vi "HO6_Generator4.vi"() -> ()   [LabVIEW 2020]
panel:
  out "XY Graph":cluster{dbl[], dbl[]}(graph)
  out "Waveform Graph":waveform(dbl)[](graph)
  out "Exceed Low Threshold":bool
  out "Exceed High Threshold":bool
  out "High Threshold":dbl
  out "Low Threshold":dbl
  in  "stop":bool
  out "Strip Chart":T1(graph)
  in  "Max":dbl=500.0
  in  "Min":dbl=100.0
  out "When slope is >0, than it's green.":bool
  out "Current Overall average":dbl
  out "Biggest/Smallest value":T2 {"Big time" format="%<%.3X>T"}
  in  "Averaged Points":i16=5 min=1 max=1024 step=1
  in  "?":bool
  in  "Mode":bool
  out "?":enum32{"Iterations", "Timed"}(tab)
  out "Iterations Remaining":i32=15
  in  "Iterations to run":i32=10 min=1 step=1
  in  "Time to run (s)":dbl=15.0
  in  "Delay (ms)":i16=500
  out "Countdown (s)":dbl caption="Elapsed Time (s)"
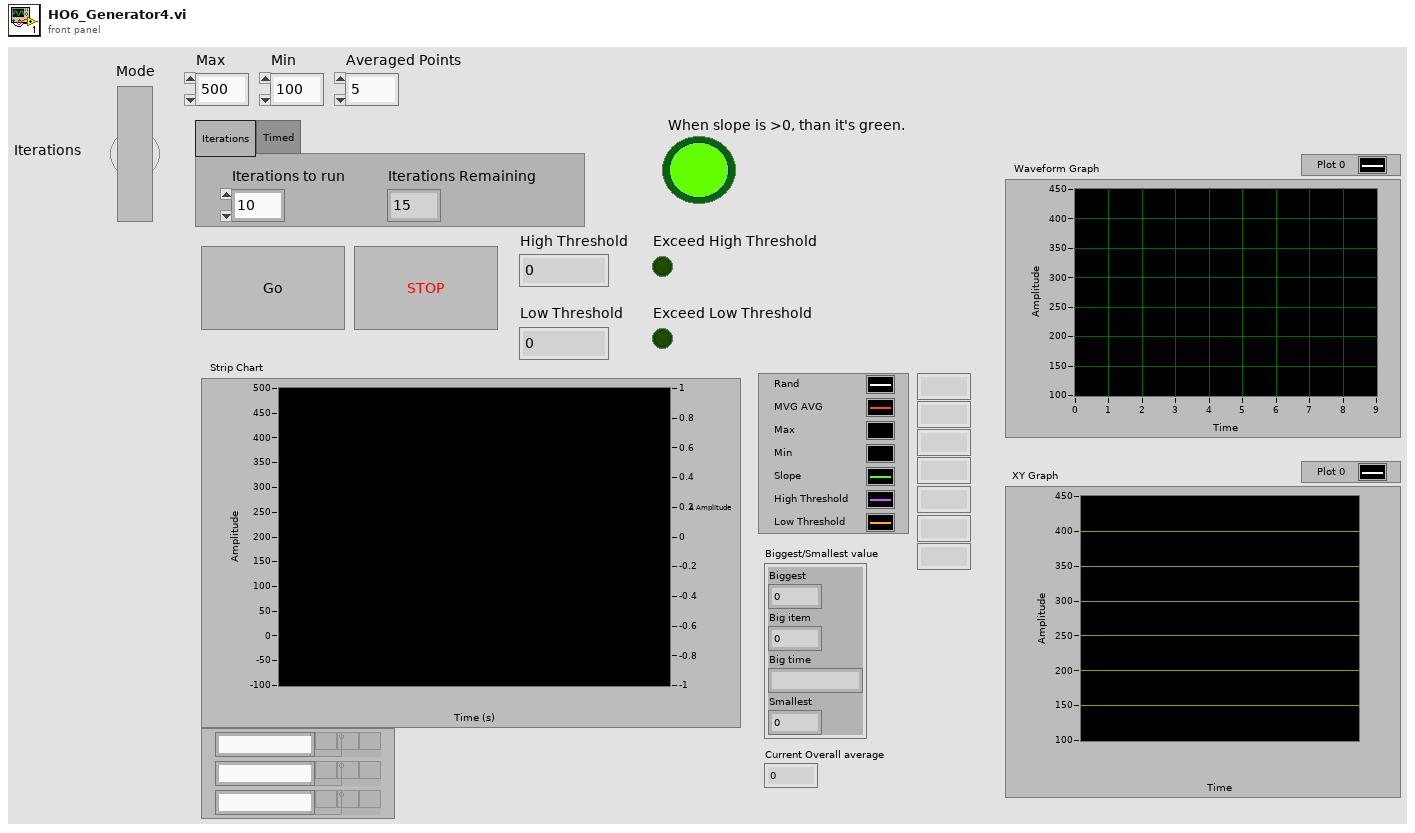
[diagram p1: front panel]
types:
  T1 = cluster{"Double":dbl, dbl, "Max":dbl, "Min":dbl, "Theta (degree)":dbl, dbl, dbl}
  T2 = cluster{"Biggest":dbl, "Big item":i32, "Big time":timestamp, "Smallest":dbl}
  T3 = cluster{"Double":dbl, dbl, "Max":dbl, "Min":dbl, "Theta (degree)":dbl, dbl, dbl}[]
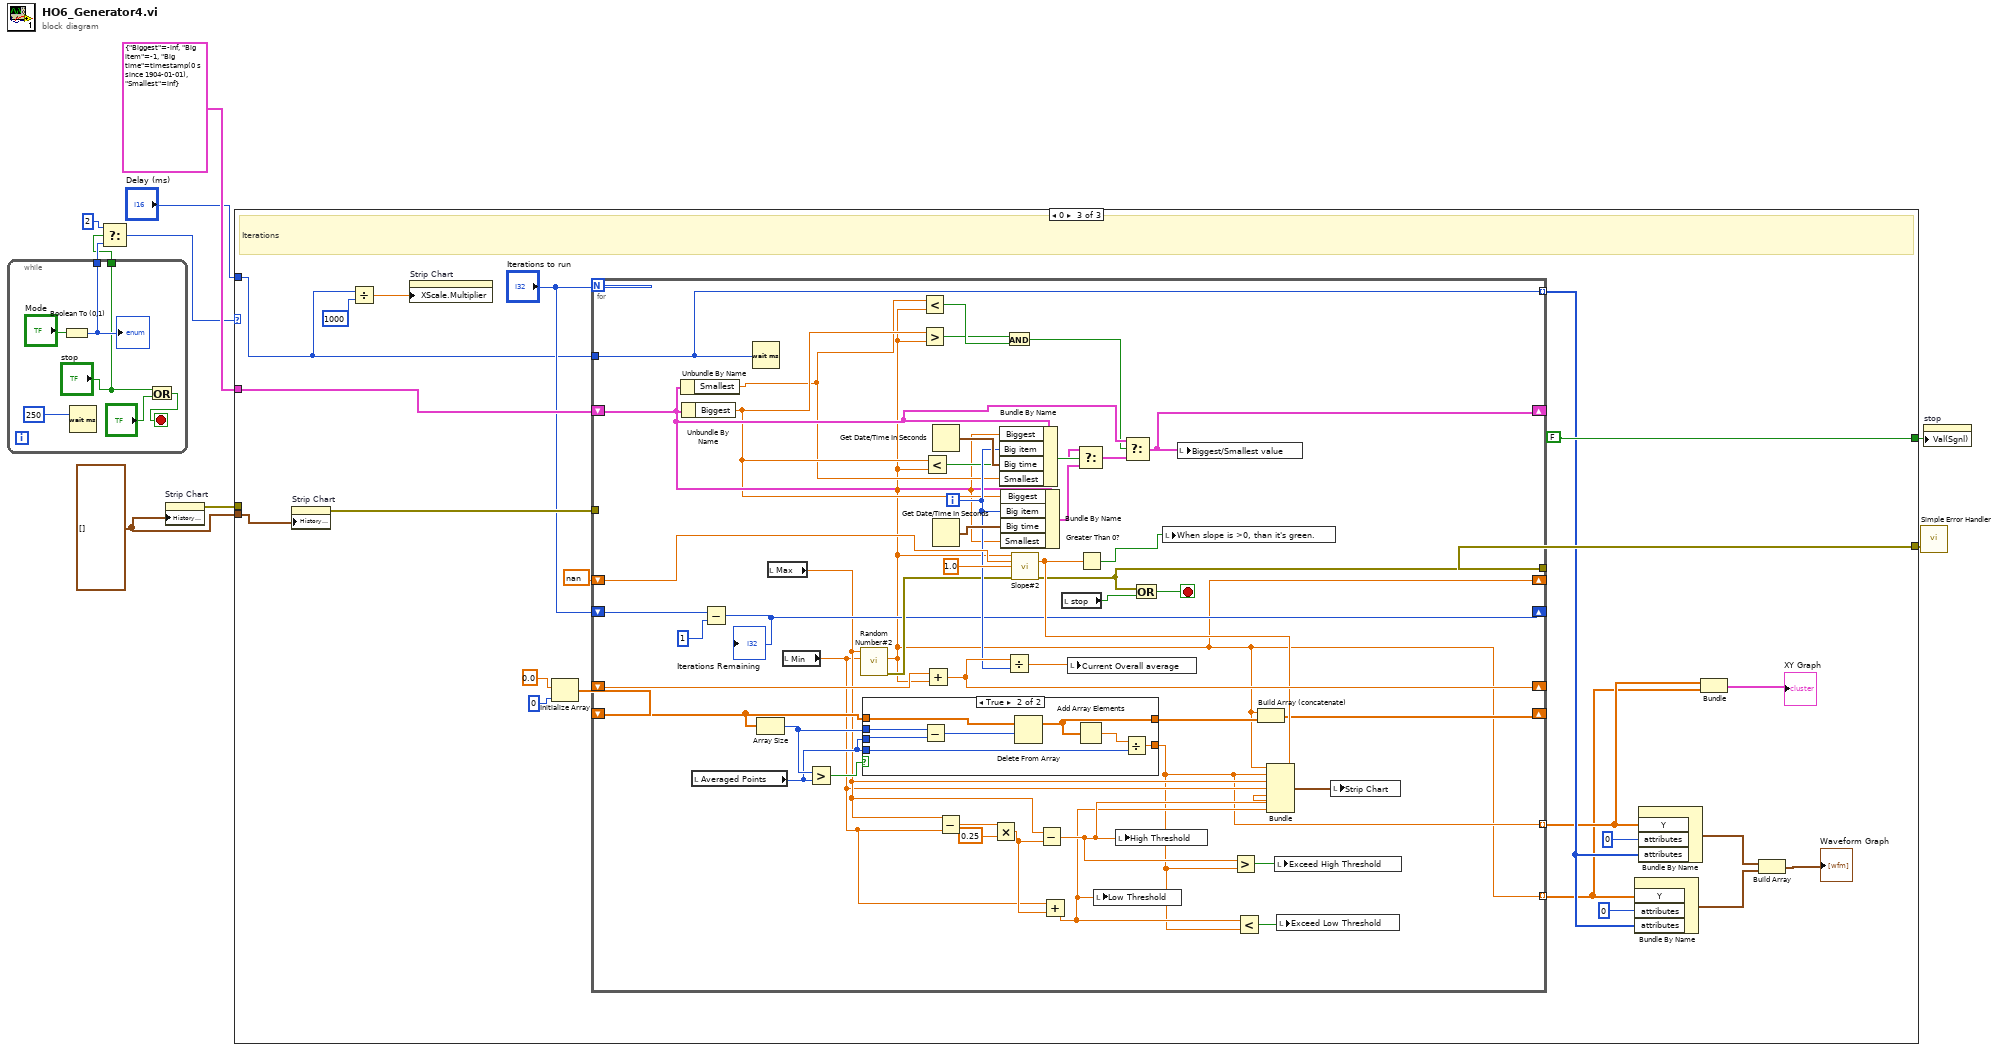
[diagram p0: block diagram]
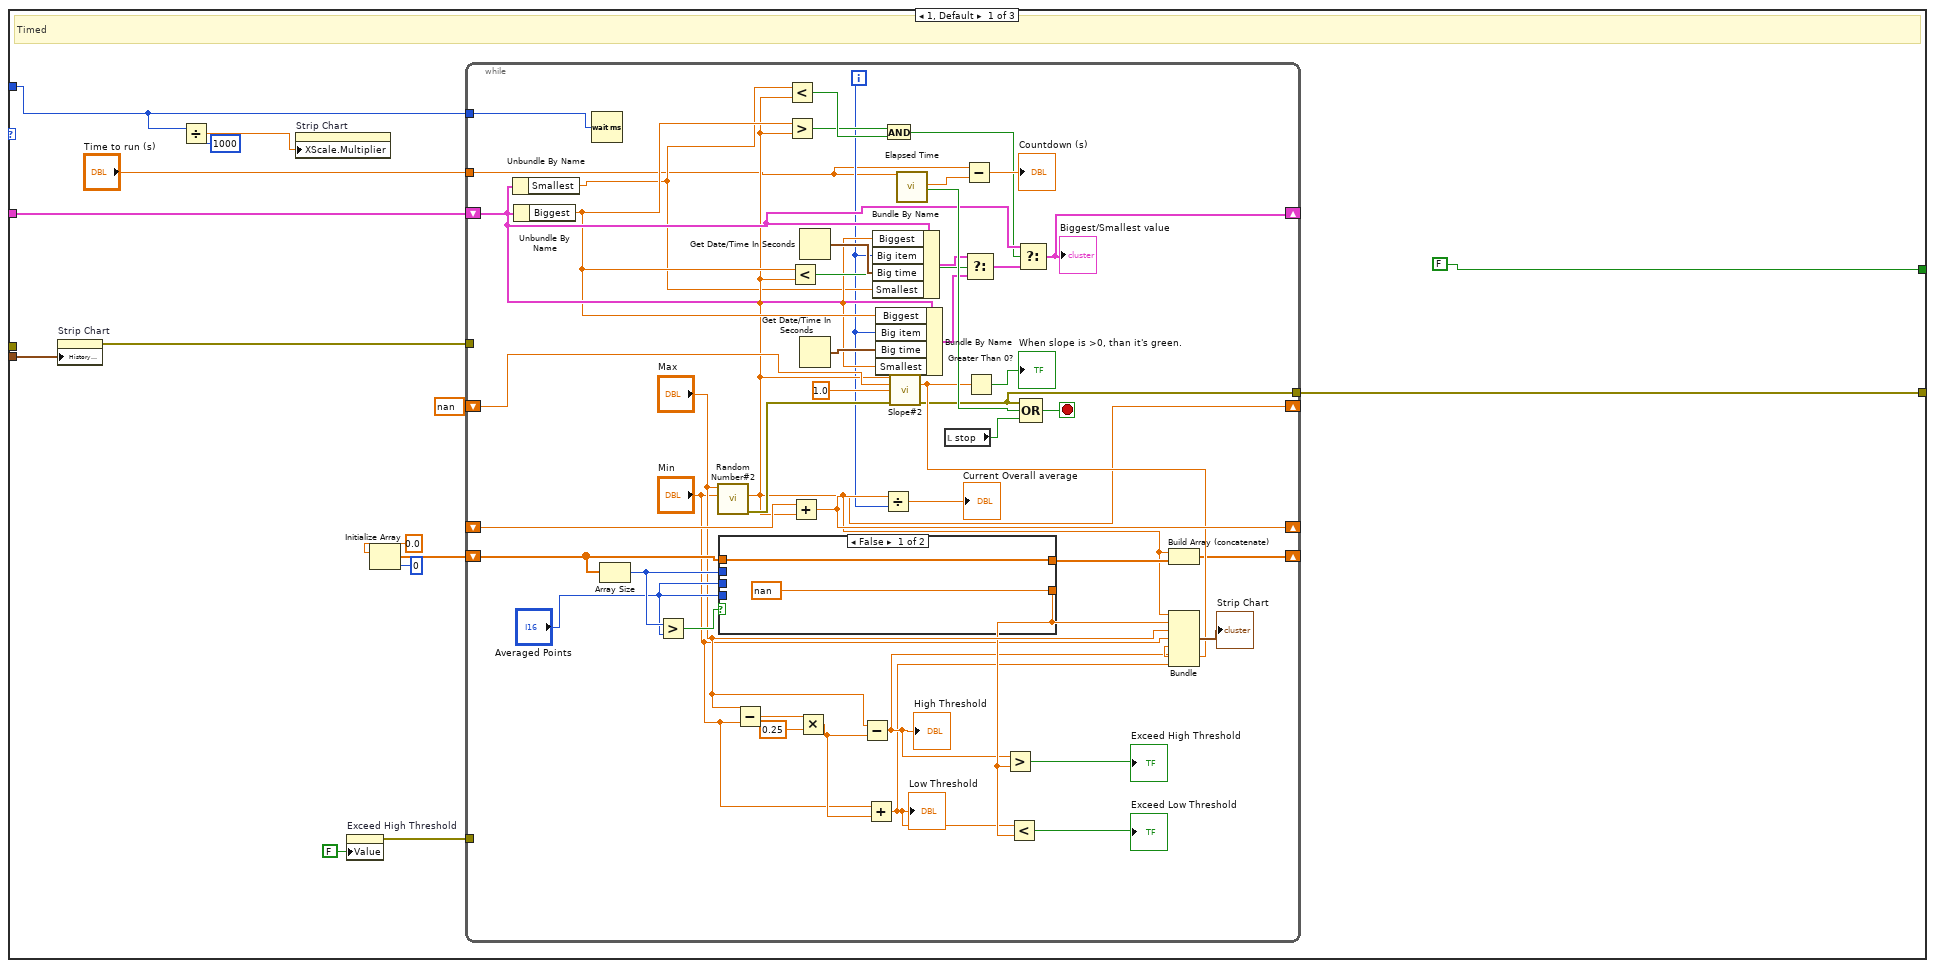
[diagram p2: hidden frame]
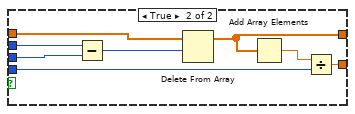
[diagram p3: hidden frame]
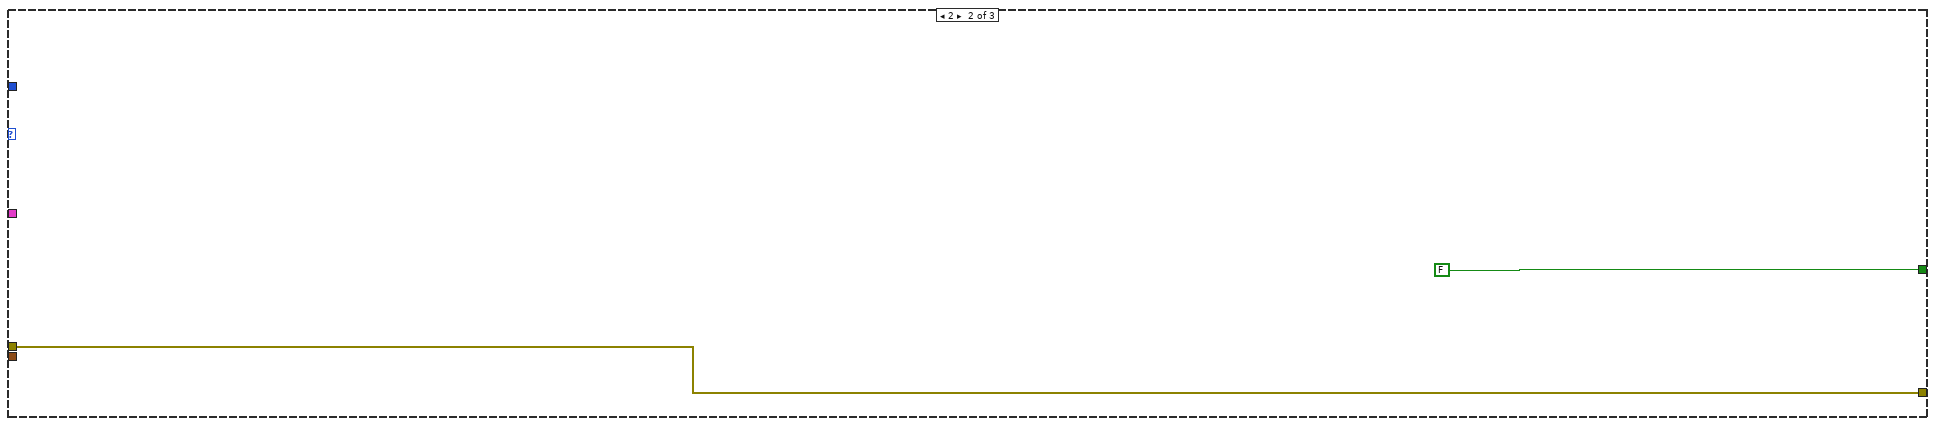
[diagram p4: hidden frame]
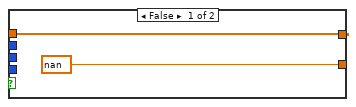
[diagram p5: hidden frame]
diagram:
  w1 = T3 [] ("History Data")
  n1 = while {
    tunnel: [w12] -> w7
    tunnel: ["stop"] -> w3
    stop <- w14 stop-if-true
    n2 = Boolean To (0,1)(Boolean="Mode") -> (0, 1=w12:i16)
    "?" <- w12
    n3 = Wait (ms)(milliseconds to wait=u32 250 ("millisecond timer value")) -> ()  [unwired: 1 out]
    n4 = Or(x="stop", y="?") -> (x .or. y?=w14:bool)
  }
  n5 = Select(t=i16 2, s=w3, f=w7) -> (s? t:f=w6:i16)
  n6 = property on="Strip Chart" class="WFChart (strict)"("History Data"=w1) -> (error out=w4:errorcluster)  [unwired: 2 in, 1 out]
  n7 = case shown="0" w6 {
    tunnel: T2 {"Biggest"=-inf, "Big item"=-1, "Big time"=timestamp(0 s since 1904-01-01), "Smallest"=inf} -> [w26 _ w109]
    tunnel: w1 -> [w25 _ w107]
    tunnel: [w24 w91 w108] -> w9
    tunnel: "Delay (ms)" -> [w23 _ w104]
    tunnel: w4 -> [_ w91 _]
    tunnel: [FALSE FALSE FALSE] -> w2
    frame 1, Default {
      # "Timed"
      n8 = property on="Strip Chart" class="WFChart (strict)"("History Data"=w25) -> (error out=w30:errorcluster)  [unwired: 2 in, 1 out]
      n9 = Divide(x=w23, y=i16 1000) -> (x/y=w20:dbl)
      n10 = property on="Strip Chart" class="WFChart (strict)"("XScale.Multiplier"=w20) -> ()  [unwired: 2 in, 2 out]
      n11 = property on="Exceed High Threshold" class="Bool (strict)"("Value"=FALSE ("Exceed High Threshold")) -> (error out=w17:errorcluster)  [unwired: 2 in, 1 out]
      n12 = Initialize Array(0.0 ("element"), 0 ("dimension size")) -> (w31:dbl[])
      n13 = while {
        tunnel: w30 -> [_]
        shift-right: [w75] -> _
        shift-left: _ -> [w76]
        tunnel: [w68] -> w24
        shift-right: [w50] -> _
        shift-left: nan -> [w67]
        shift-right: [w65] -> _
        shift-left: w26 -> [w62]
        shift-right: [w56] -> _
        shift-left: w31 -> [w54]
        tunnel: "Time to run (s)" -> [w43]
        tunnel: w23 -> [w44]
        tunnel: w17 -> [_]
        i -> [w45]
        stop <- w74 stop-if-true
        n14 = Unbundle By Name(w62) -> ("Smallest"=w49:dbl)
        n15 = Unbundle By Name(w62) -> ("Biggest"=w51:dbl)
        n16 = Wait (ms)(milliseconds to wait=w44) -> ()  [unwired: 1 out]
        n17 = Array Size(array=w54) -> (size(s)=w53:i32)
        n18 = Greater?(x=w53, y="Averaged Points") -> (0:w55:bool)
        n19 = call "Random Number#2.vi"("Maximum"="Max", "Minimum"="Min") -> ("Double"=w50:dbl, "error out"=w69:errorcluster)  [unwired: 4 in, 2 out]
        n20 = case shown="False" w55 {
          tunnel: w54 -> [w81 w89]
          tunnel: w53 -> [_ w87]
          tunnel: "Averaged Points" -> [_ w86]
          tunnel: "Averaged Points" -> [_ w85]
          tunnel: [nan w84] -> w37
          tunnel: [w81 w82] -> w52
          frame False {
          }
          frame True {
            n21 = Subtract(x=w87, y=w86) -> (x-y=w88:i32)
            n22 = Delete From Array(array=w89, length=w88) -> (array with subset deleted=w82:dbl[])  [unwired: 1 in, 1 out]
            n23 = Add Array Elements(numeric array=w82) -> (sum=w83:dbl)
            n24 = Divide(x=w83, y=w85) -> (x/y=w84:dbl)
          }
        }
        n25 = Subtract(x="Max", y="Min") -> (x-y=w41:dbl)
        n26 = Less?(x=w49, y=w50) -> (x < y?=w61:bool)
        n27 = Greater?(x=w51, y=w50) -> (0:w58:bool)
        n28 = Less?(x=w51, y=w50) -> (x < y?=w57:bool)
        n29 = Add(x=w76, y=w50) -> (x+y=w75:dbl)
        n30 = Multiply(x=w41, y=0.25) -> (x*y=w39:dbl)
        n31 = Get Date/Time In Seconds() -> (seconds since 1Jan1904=w64:timestamp)
        n32 = Get Date/Time In Seconds() -> (seconds since 1Jan1904=w63:timestamp)
        n33 = Subtract(x="Max", y=w39) -> (x-y=w35:dbl)
        "High Threshold" <- w35
        n34 = Add(x="Min", y=w39) -> (x+y=w34:dbl)
        "Low Threshold" <- w34
        n35 = Bundle By Name(cluster=w62, "Biggest"=w50, "Big item"=w45, "Big time"=w64, "Smallest"=w49) -> (w47:T2)
        n36 = Bundle By Name(cluster=w62, "Biggest"=w51, "Big item"=w45, "Big time"=w63, "Smallest"=w50) -> (w48:T2)
        n37 = Divide(x=w75, y=w45) -> (x/y=→"Current Overall average":dbl)
        n38 = And(x=w58, y=w61) -> (x .and. y?=w60:bool)
        n39 = call "Slope#2.vi"("Y2"=w50, "Y1"=w67, "X2 (1)"=1.0, "error in (no error)"=w69) -> ("Theta (degree)"=w70:dbl, "error out"=w68:errorcluster)  [unwired: 8 in, 2 out]
        n40 = call "Elapsed Time"("Time Target (s)"=w43) -> ("Elapsed Time (s)"=w72:dbl, "Time has Elapsed"=w73:bool)  [unwired: 11 in, 6 out]
        n41 = local read "stop"() -> (w42:bool)
        n42 = Subtract(x=w43, y=w72) -> (x-y=→"Countdown (s)":dbl)
        n43 = Select(t=w47, s=w57, f=w48) -> (s? t:f=w59:T2)
        n44 = Greater Than 0?(x=w70) -> (x > 0?=→"When slope is >0, than it's green.":bool)
        n45 = Greater?(x=w35, y=w37) -> (0:→"Exceed High Threshold":bool)
        n46 = Less?(x=w34, y=w37) -> (x < y?=→"Exceed Low Threshold":bool)
        n47 = Select(t=w62, s=w60, f=w59) -> (s? t:f=w65:T2)
        "Biggest/Smallest value" <- w65
        n48 = Compound Arithmetic op=OR(w68, w73, w42) -> (w74:bool)
        n49 = Build Array (concatenate)(w50, w52) -> (w56:dbl[])
        n50 = Bundle("Double"=w50, w37, "Max"="Max", "Min"="Min", "Theta (degree)"=w70, w35, w34) -> (→"Strip Chart":T1)  [unwired: 1 in]
      }
    }
    frame 2 {
    }
    frame 0 {
      # "Iterations"
      n51 = property on="Strip Chart" class="WFChart (strict)"("History Data"=w107) -> (error out=w106:errorcluster)  [unwired: 2 in, 1 out]
      n52 = Divide(x=w104, y=i16 1000) -> (x/y=w102:dbl)
      n53 = property on="Strip Chart" class="WFChart (strict)"("XScale.Multiplier"=w102) -> ()  [unwired: 2 in, 2 out]
      n54 = Initialize Array(0.0 ("element"), 0 ("dimension size")) -> (w113:dbl[])
      n55 = for {
        N: "Iterations to run" -> [_]
        shift-right: [w159] -> _
        shift-left: _ -> [w160]
        tunnel: [w128] -> w108
        shift-right: [w114] -> _
        shift-left: nan -> [w157]
        shift-right: [w137] -> _
        shift-left: w109 -> [w152]
        shift-right: [w146] -> _
        shift-left: w113 -> [w144]
        tunnel: w106 -> [_]
        shift-right: [w129] -> _
        shift-left: "Iterations to run" -> [w131]
        tunnel: w104 -> [w115]
        tunnel: [w116] -> w94 mode=indexing
        tunnel: [w115] -> w98 mode=indexing
        tunnel: [w114] -> w93 mode=indexing
        i -> [w153]
        stop <- w126 stop-if-true
        n56 = Unbundle By Name(w152) -> ("Smallest"=w140:dbl)
        n57 = Unbundle By Name(w152) -> ("Biggest"=w141:dbl)
        n58 = local read "Averaged Points"() -> (w134:i16)
        n59 = Subtract(x=w131, y=1) -> (x-y=w129:i32)
        "Iterations Remaining" <- w129
        n60 = Wait (ms)(milliseconds to wait=w115) -> ()  [unwired: 1 out]
        n61 = Array Size(array=w144) -> (size(s)=w143:i32)
        n62 = local read "Max"() -> (w123:dbl)
        n63 = local read "Min"() -> (w121:dbl)
        n64 = Greater?(x=w143, y=w134) -> (0:w145:bool)
        n65 = call "Random Number#2.vi"("Maximum"=w123, "Minimum"=w121) -> ("Double"=w114:dbl, "error out"=w132:errorcluster)  [unwired: 4 in, 2 out]
        n66 = case shown="True" w145 {
          tunnel: w144 -> [w162 w170]
          tunnel: w143 -> [_ w168]
          tunnel: w134 -> [_ w167]
          tunnel: w134 -> [_ w166]
          tunnel: [nan w165] -> w116
          tunnel: [w162 w163] -> w142
          frame False {
          }
          frame True {
            n67 = Subtract(x=w168, y=w167) -> (x-y=w169:i32)
            n68 = Delete From Array(array=w170, length=w169) -> (array with subset deleted=w163:dbl[])  [unwired: 1 in, 1 out]
            n69 = Add Array Elements(numeric array=w163) -> (sum=w164:dbl)
            n70 = Divide(x=w164, y=w166) -> (x/y=w165:dbl)
          }
        }
        n71 = Less?(x=w140, y=w114) -> (x < y?=w151:bool)
        n72 = Greater?(x=w141, y=w114) -> (0:w148:bool)
        n73 = Less?(x=w141, y=w114) -> (x < y?=w147:bool)
        n74 = Add(x=w160, y=w114) -> (x+y=w159:dbl)
        n75 = Get Date/Time In Seconds() -> (seconds since 1Jan1904=w155:timestamp)
        n76 = Get Date/Time In Seconds() -> (seconds since 1Jan1904=w154:timestamp)
        n77 = Subtract(x=w123, y=w121) -> (x-y=w125:dbl)
        n78 = Multiply(x=w125, y=0.25) -> (x*y=w122:dbl)
        n79 = Bundle By Name(cluster=w152, "Biggest"=w114, "Big item"=w153, "Big time"=w155, "Smallest"=w140) -> (w138:T2)
        n80 = Bundle By Name(cluster=w152, "Biggest"=w141, "Big item"=w153, "Big time"=w154, "Smallest"=w114) -> (w139:T2)
        n81 = Divide(x=w159, y=w153) -> (x/y=w136:dbl)
        n82 = And(x=w148, y=w151) -> (x .and. y?=w150:bool)
        n83 = call "Slope#2.vi"("Y2"=w114, "Y1"=w157, "X2 (1)"=1.0, "error in (no error)"=w132) -> ("Theta (degree)"=w158:dbl, "error out"=w128:errorcluster)  [unwired: 8 in, 2 out]
        n84 = Subtract(x=w123, y=w122) -> (x-y=w118:dbl)
        n85 = Add(x=w121, y=w122) -> (x+y=w117:dbl)
        n86 = local read "stop"() -> (w127:bool)
        n87 = local write "Current Overall average"(w136) -> ()
        n88 = Select(t=w138, s=w147, f=w139) -> (s? t:f=w149:T2)
        n89 = Greater Than 0?(x=w158) -> (x > 0?=w135:bool)
        n90 = local write "Low Threshold"(w117) -> ()
        n91 = local write "High Threshold"(w118) -> ()
        n92 = Select(t=w152, s=w150, f=w149) -> (s? t:f=w137:T2)
        n93 = Compound Arithmetic op=OR(w128, w127) -> (w126:bool)
        n94 = local write "When slope is >0, than it's green."(w135) -> ()
        n95 = local write "Biggest/Smallest value"(w137) -> ()
        n96 = Greater?(x=w118, y=w116) -> (0:w120:bool)
        n97 = Less?(x=w117, y=w116) -> (x < y?=w119:bool)
        n98 = Build Array (concatenate)(w114, w142) -> (w146:dbl[])
        n99 = Bundle("Double"=w114, w116, "Max"=w123, "Min"=w121, "Theta (degree)"=w158, w118, w117) -> (w133:T1)  [unwired: 1 in]
        n100 = local write "Exceed High Threshold"(w120) -> ()
        n101 = local write "Exceed Low Threshold"(w119) -> ()
        n102 = local write "Strip Chart"(w133) -> ()
      }
      n103 = Bundle By Name("Y"=w93, "attributes"=0, "attributes"=w98) -> (w96:waveform(dbl))  [unwired: 1 in]
      n104 = Bundle By Name("Y"=w94, "attributes"=0, "attributes"=w98) -> (w97:waveform(dbl))  [unwired: 1 in]
      n105 = Bundle(w94, w93) -> (→"XY Graph":cluster{dbl[], dbl[]})  [unwired: 1 in]
      n106 = Build Array(w97, w96) -> (→"Waveform Graph":waveform(dbl)[])
    }
  }
  n107 = call <vilib>:"Simple Error Handler.vi"("error in (no error)"=w9) -> ()  [unwired: 4 in, 5 out]
  n108 = property on="stop" class="Bool (strict)"("Val(Sgnl)"=w2) -> ()  [unwired: 2 in, 2 out]
